vi "3KantVip_SubVI.vi"() -> ()   [LabVIEW 2018]
panel:
  out "Direction":bool
  out "Enable 3":bool
  out "Enable 2":bool
  out "Enable 1":bool
  in  "stop":bool
  in  "BUND!":bool
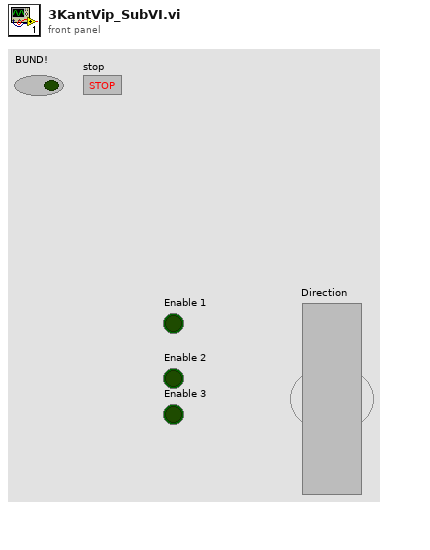
[diagram p1: front panel]
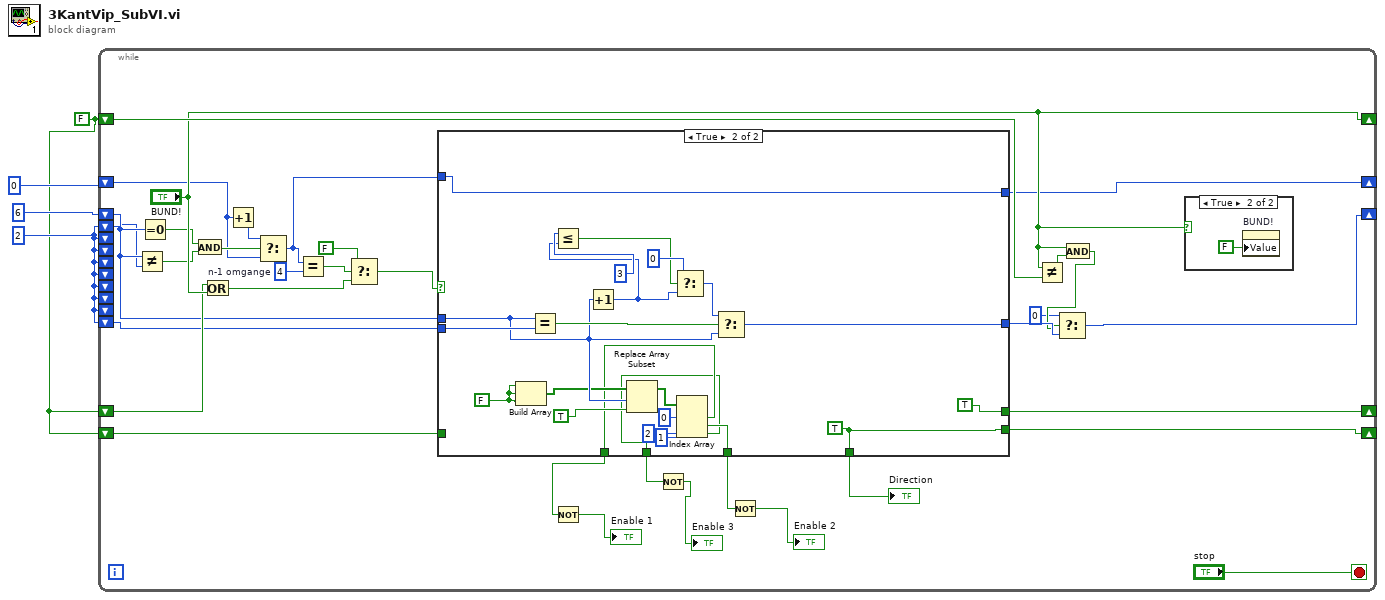
[diagram p0: block diagram]
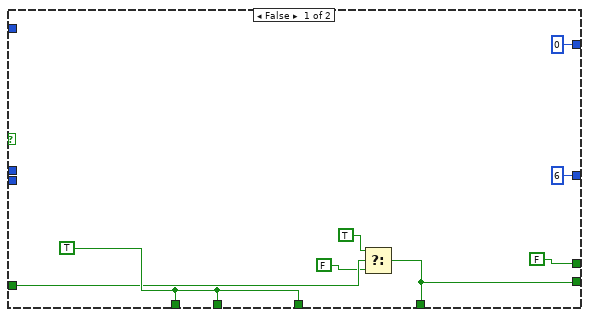
[diagram p3: hidden frame]
diagram:
  w1 = FALSE ("BUND!")
  w3 = 2
  n1 = while {
    shift-right: [w36] -> _
    shift-left: 6 -> [w27]
    shift-left: w3 -> [w26]
    shift-left: w3 -> [_]
    shift-left: w3 -> [_]
    shift-left: w3 -> [_]
    shift-left: w3 -> [_]
    shift-left: w3 -> [_]
    shift-left: w3 -> [_]
    shift-left: w3 -> [_]
    shift-left: w3 -> [w28]
    shift-right: ["BUND!"] -> _
    shift-left: w1 -> [w34]
    shift-right: [w30] -> _
    shift-left: w1 -> [w29]
    shift-right: [w20] -> _
    shift-left: 0 -> [w21]
    shift-right: [w11] -> _
    shift-left: w1 -> [w12]
    stop <- "stop" stop-if-true
    w18 = 4  # n-1 omgange
    n2 = Not Equal?(x=w27, y=w26) -> (x != y?=w24:bool)
    n3 = Equal To 0?(x=w27) -> (x = 0?=w25:bool)
    n4 = And(x=w25, y=w24) -> (x .and. y?=w23:bool)
    n5 = Or(x=w29, y="BUND!") -> (x .or. y?=w16:bool)
    n6 = Increment(x=w21) -> (x+1=w22:i32)
    n7 = Select(t=w22, s=w23, f=w21) -> (s? t:f=w19:i32)
    n8 = Equal?(x=w19, y=w18) -> (x = y?=w17:bool)
    n9 = Select(t=FALSE, s=w17, f=w16) -> (s? t:f=w15:bool)
    n10 = case shown="True" w15 {
      tunnel: w28 -> [_ w69]
      tunnel: w27 -> [_ w59]
      tunnel: [6 ("t") w65] -> w37
      tunnel: [FALSE TRUE ("BUND!")] -> w30
      tunnel: [0 w61] -> w20
      tunnel: w19 -> [_ w61]
      tunnel: [w44 w51] -> w9
      tunnel: [w44 w49] -> w8
      tunnel: [w44 w50] -> w5
      tunnel: [w40 w48] -> w13
      tunnel: w12 -> [w43 _]
      tunnel: [w40 w48] -> w11
      frame False {
        w44 = TRUE
        n11 = Select(t=TRUE, s=w43, f=FALSE) -> (s? t:f=w40:bool)
      }
      frame True {
        w48 = TRUE ("BUND!")
        w57 = FALSE
        n12 = Build Array(w57, w57, w57) -> (w58:bool[])
        n13 = Equal?(x=w59, y=w69) -> (x = y?=w68:bool)
        n14 = Increment(x=w59) -> (x+1=w62:i32)
        n15 = Less Or Equal?(x=3, y=w62) -> (x <= y?=w64:bool)
        n16 = Replace Array Subset(array=w58, new element=TRUE, index=w59) -> (w55:bool[])
        n17 = Select(t=0, s=w64, f=w62) -> (s? t:f=w67:i32)
        n18 = Index Array(array=w55, index #1=0 ("index"), index #2=1 ("index"), index #3=2 ("index")) -> (element #1=w51:bool, element #2=w50:bool, element #3=w49:bool)
        n19 = Select(t=w67, s=w68, f=w59) -> (s? t:f=w65:i32)
      }
    }
    "Direction" <- w13
    n20 = Not(x=w9) -> (.not. x?=→"Enable 1":bool)
    n21 = Not(x=w8) -> (.not. x?=→"Enable 3":bool)
    n22 = Not(x=w5) -> (.not. x?=→"Enable 2":bool)
    n23 = Not Equal?(x="BUND!", y=w34) -> (x != y?=w35:bool)
    n24 = And(x="BUND!", y=w35) -> (x .and. y?=w33:bool)
    n25 = Select(t=0, s=w33, f=w37) -> (s? t:f=w36:i32)
    n26 = case shown="True" "BUND!" {
      frame False {
      }
      frame True {
        n27 = property on="BUND!" class="Bool (strict)"("Value"=FALSE ("BUND!")) -> ()  [unwired: 2 in, 2 out]
      }
    }
  }
